vi "Get Config File Path For Engineer Mode.vi"(11 "error in (no error)":errorcluster) -> (4 "Config File Path":path, 15 "error out":errorcluster)   [LabVIEW 2023, in "RFFixtureCharact.Public.lvlib"]
uses:
  RFFixtureCharact.Public.lvlib
  <vilib>/regexp/Match Regular Expression.xnode
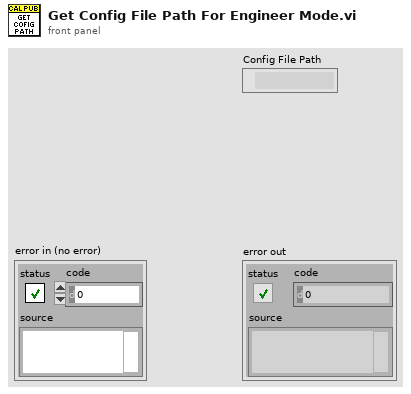
[diagram p1: front panel]
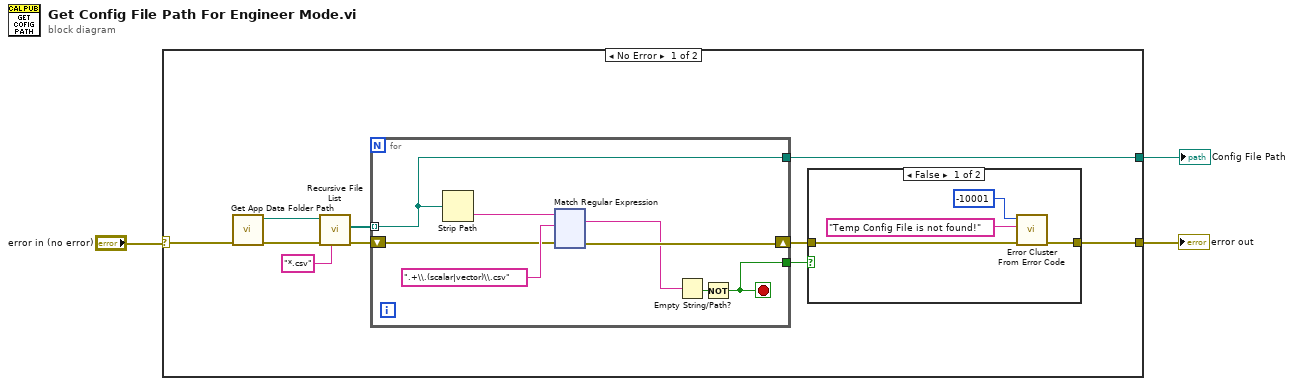
[diagram p0: block diagram]
diagram:
  n1 = case shown="No Error" "error in (no error)" {
    selector: "error in (no error)" -> [w5 w144]
    tunnel: [w12 w144] -> w2
    tunnel: [w13 _] -> w1
    frame No Error {
      n2 = call "Get App Data Folder Path.vi"("error in (no error)"=w5) -> ("error out"=w4:errorcluster, "Temp Folder Path"=w10:path)  [unwired: 9 in]
      n3 = call <vilib>:"Recursive File List.vi"("pattern"="*.csv", "error in (no error)"=w4, "Folder Path"=w10) -> ("error out"=w9:errorcluster, "All Files in Dir"=w8:path[])  [unwired: 4 in, 3 out]
      n4 = for {
        tunnel: w8 -> [w22] mode=indexing
        shift-right: [w23] -> w6
        shift-left: w9 -> [w25]
        tunnel: [w22] -> w13
        tunnel: [w19] -> w7
        stop <- w19 stop-if-true
        n5 = Strip Path(path=w22) -> (name=w24:string)  [unwired: 1 out]
        n6 = xnode "Match Regular Expression"("input string"=w24, "regular expression"=".+\\.(scalar|vector)\\.csv", "error in"=w25) -> ("whole match"=w21:string, "error out"=w23:errorcluster)  [unwired: 3 in, 3 out]
        n7 = Empty String/Path?(string/path=w21) -> (empty?=w20:bool)
        n8 = Not(x=w20) -> (.not. x?=w19:bool)
      }
      n9 = case shown="False" w7 {
        tunnel: [w16 w18] -> w12
        tunnel: w6 -> [w17 w18]
        frame False {
          n10 = call <vilib>:"Error Cluster From Error Code.vi"("error in (no error)"=w17, "error message (\"\")"="Temp Config File is not found!" ("error source (\" \")"), "error code (0)"=-10001 ("error code (no error:0)")) -> ("error out"=w16:errorcluster)  [unwired: 6 in]
        }
        frame True {
        }
      }
    }
    frame Error {
    }
  }
  "error out" <- w2
  "Config File Path" <- w1
